vi "Parse DBL Array.vi"(6 "Seperator":string=",", 8 "error in":errorcluster, 9 "Input <JSON>":string, 10 "csv string":string, 11 "Simple CSV Parser in":refnum<class "Simple CSV Parser.lvclass">) -> (0 "error out":errorcluster, 2 "DBL Array":dbl[](array[numeric]), 3 "Simple CSV Parser out":refnum<class "Simple CSV Parser.lvclass">)   [LabVIEW 2020, in "Simple CSV Parser.lvclass"]
uses:
  Simple CSV Parser.lvclass
  Simple CSV Parser.lvclass/Simple CSV Parser.ctl
  38e74525-b6bf-4b5c-91f2-ddc5eb39488b.vi
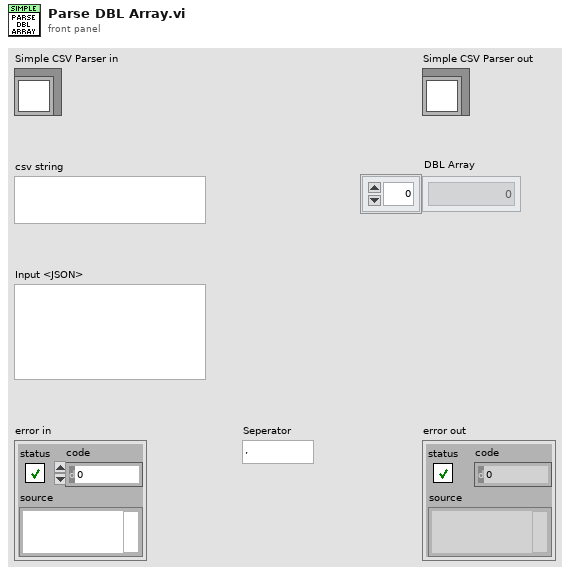
[diagram p1: front panel]
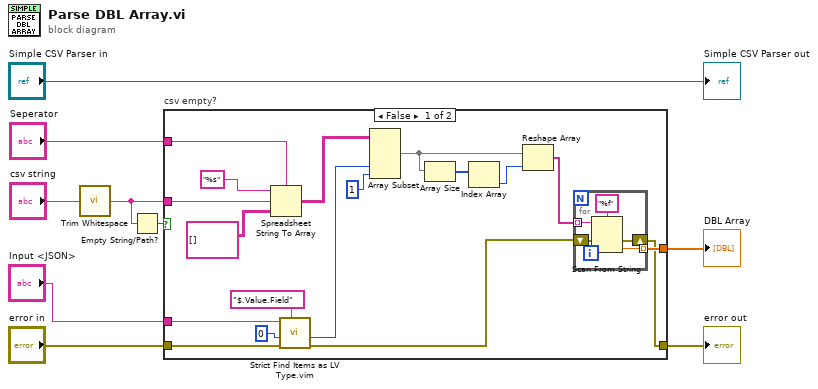
[diagram p0: block diagram]
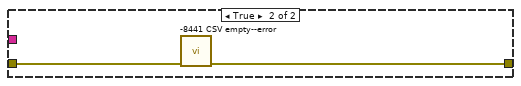
[diagram p2: hidden frame]
diagram:
  n1 = call <vilib>:"Trim Whitespace.vi"("string"="csv string") -> ("trimmed string"=w1:string)  [unwired: 1 in]
  n2 = Empty String/Path?(string/path=w1) -> (empty?=w3:bool)
  n3 = case "csv empty?" shown="False" w3 {
    tunnel: w1 -> [w19 _]
    tunnel: [w18 _] -> w8
    tunnel: "Seperator" -> [w17 _]
    tunnel: "error in" -> [w16 w34]
    tunnel: "Input <JSON>" -> [w15 _]
    tunnel: [w10 w33] -> w4
    frame False {
      n4 = Spreadsheet String To Array(delimiter (Tab)=w17, format string="%s", spreadsheet string=w19, array type (2D Dbl)=string[][] []) -> (array=w25:string[][])
      n5 = call "Strict Find Items as LV Type.vim"("$Path or Item Name"="$.Value.Field", "error in"=w16, "Data Type and Default Value"=0, "<JSON>"=w15) -> ("error out"=w11:errorcluster, "Data out"=w12:i32)  [unwired: 5 in, 1 out]
      n6 = Array Subset(array=w25, index (col)=w12, length (col)=1 ("length")) -> (w23:string[][])  [unwired: 2 in]
      n7 = Array Size(array=w23) -> (size(s)=w22:i32[])
      n8 = Index Array(array=w22) -> (element=w21:i32)  [unwired: 1 in]
      n9 = Reshape Array(w23, w21) -> (w20:string[])
      n10 = for {
        tunnel: w20 -> [w32] mode=indexing
        tunnel: [w31] -> w18 mode=indexing
        shift-right: [w28] -> w10
        shift-left: w11 -> [w29]
        n11 = Scan From String(format string="%f", input string=w32, error in=w29) -> (error out=w28:errorcluster, output 1=w31:dbl)  [unwired: 2 in, 2 out]
      }
    }
    frame True {
      n12 = call "-8441 CSV empty--error.vi"("error in"=w34) -> ("error out"=w33:errorcluster)  [unwired: 10 in]
    }
  }
  "error out" <- w4
  "DBL Array" <- w8
  "Simple CSV Parser out" <- "Simple CSV Parser in"
